vi "Sensor - Find theta and position - shih.vi"() -> ()   [LabVIEW 2016]
uses:
  Classes/Controllers/Motion/Copy of Motion Folder/Motion.lvclass
  Classes/Controllers/Camera/Copy of Controller Folder/Controller.lvclass
panel:
  out "Type B rotation error":dbl format="%#_8e"
  out "Type B Y error":dbl format="%#_8g"
  out "Type B X error":dbl format="%#_8g"
  out "Type A rotation error":dbl format="%#_8e"
  out "Type A Y error":dbl format="%#_8g"
  out "Type A X error":dbl format="%#_8g"
  in  "position A":dbl[](array[numeric])=[450.0333, 1074.4422, 78.966399, 0.019289062] format="%#_10g"
  in  "Boolean":bool
  out "HDI/sesnor array":bool[](array[boolean])
  out "type a/b array":bool[](array[boolean])
  in  "C 2":dbl[](array[numeric])=[322.268517526742, 1153.5721313313948, 79.00539576014785, 0.01961841234863117] format="%#_10g"
  in  "B 2":dbl[](array[numeric])=[300.2655109951287, 1153.8313815706124, 79.00573186765678, 0.019288904062814086] format="%#_10g"
  in  "position A 2":dbl[](array[numeric])=[299.0519921586575, 1052.343019098103, 79.00564961071272, 0.019294304149470937] format="%#_10g"
  in  "C":dbl[](array[numeric])=[475.67567, 1203.3475, 78.955395, 0.019618489] format="%#_10g"
  in  "B":dbl[](array[numeric])=[451.38655, 1203.5959, 78.956401, 0.019289062] format="%#_10g"
  in  "position A 4":dbl[](array[numeric])=[299.0519921586575, 1052.343019098103, 79.00564961071272, 0.019294304149470937] format="%#_10g"
  in  "B 4":dbl[](array[numeric])=[300.2655109951287, 1153.8313815706124, 79.00573186765678, 0.019288904062814086] format="%#_10g"
  in  "C 4":dbl[](array[numeric])=[322.268517526742, 1153.5721313313948, 79.00539576014785, 0.01961841234863117] format="%#_10g"
  in  "position A 3":dbl[](array[numeric])=[450.75355, 1073.8809, 78.571159, 0.019294304149470937] format="%#_10g"
  in  "B 3":dbl[](array[numeric])=[452.11281, 1203.3722, 78.624175, 0.019288904062814086] format="%#_10g"
  in  "C 3":dbl[](array[numeric])=[474.11351, 1203.144, 78.625406, 0.01961841234863117] format="%#_10g"
  in  "Type A/ Type B":bool
  in  "HDI / Sensor":bool
  out "the copy array":dbl[](array[numeric]) format="%#_8g"
  out "buttom right C":dbl[](array[numeric]) format="%#_8g"
  out "X position":dbl[](array[numeric]) format="%#_8g"
  out "Yposition":dbl[](array[numeric]) format="%#_8g"
  out "A C center point":dbl[](array[numeric]) format="%#_8g"
  out "counting":dbl
  out "rotation":dbl[](array[numeric]) format="%#_8g"
  in  "Parking position":dbl[](array[numeric])=[625.0, 625.0, 0.0, 0.01]
  in  "Stop":bool
  in  "DO measurement":bool=TRUE
  out "buttom left B":dbl[](array[numeric]) format="%#_8g"
  out "upper left A":dbl[](array[numeric]) format="%#_8g"
  out "r-phi":dbl[](array[numeric])
  out "A B center point":dbl[](array[numeric])
  # "HDI"
  # "type A"
  # "Sensor"
  # "type B"
  # "type A"
  # "type B"
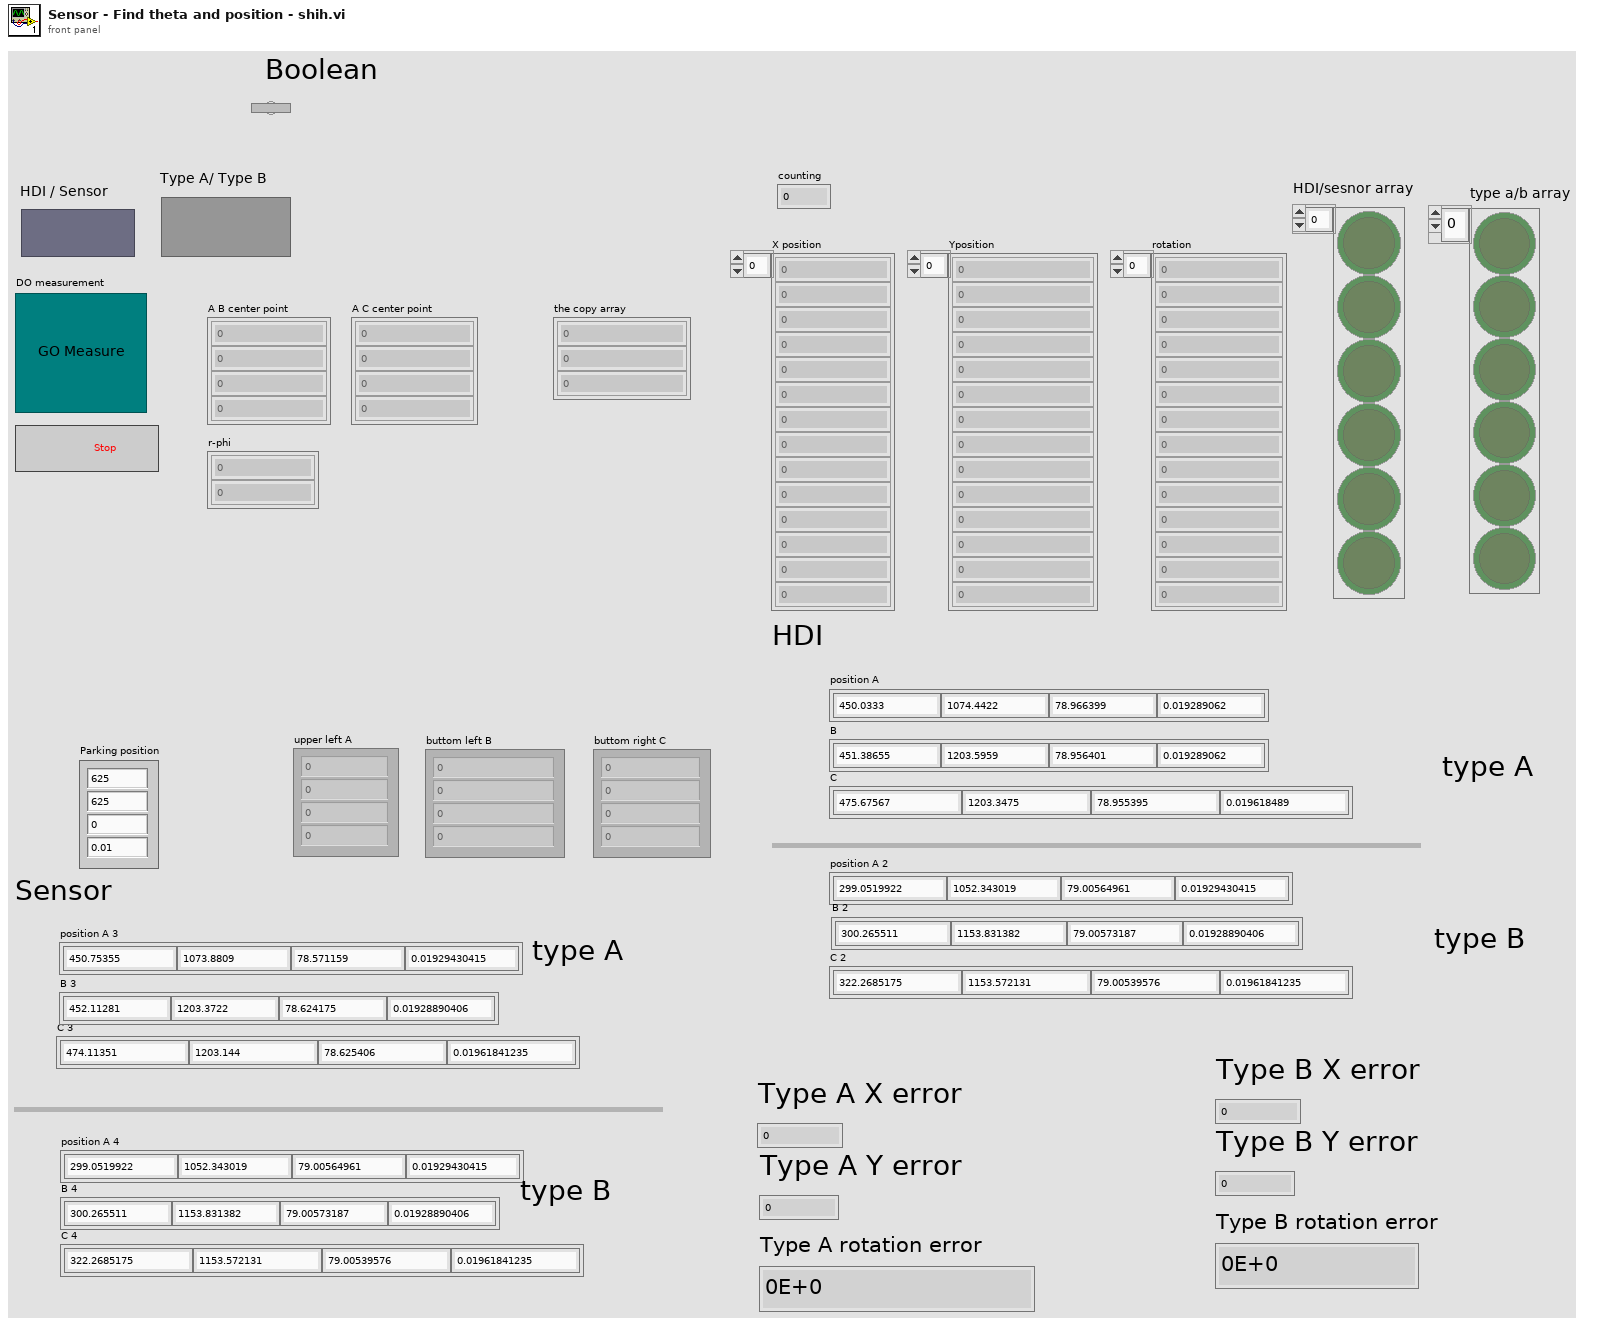
[diagram p1: front panel]
types:
  T1 = typedef "Controller.lvclass/Controllers.ctl" = cluster{"Copy of Motion.lvclass":refnum<class "Motion.lvclass">, "Copy of I-O.lvclass":refnum<class "I-O.lvclass">, "Copy of Dispenser.lvclass":refnum<class "Dispenser.lvclass">}
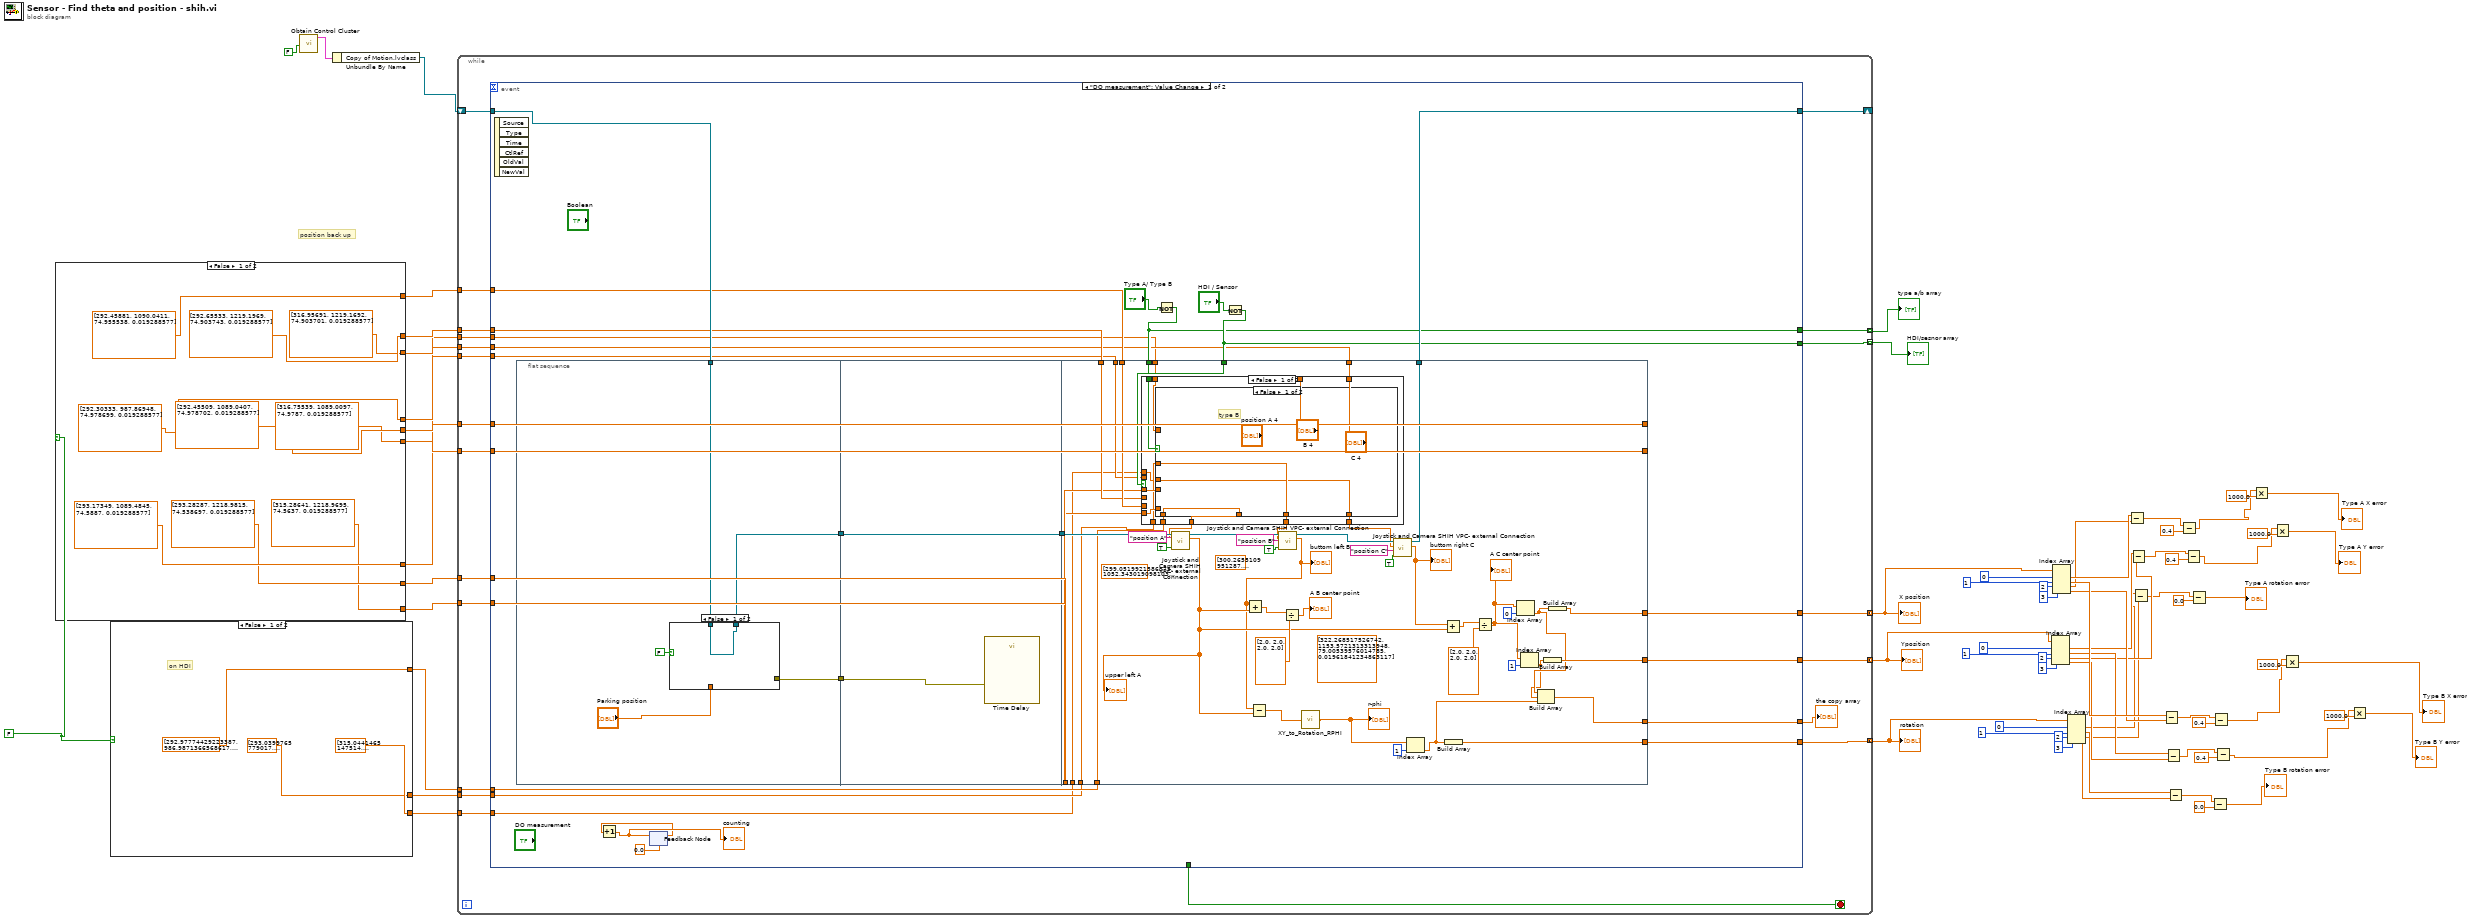
[diagram p0: block diagram]
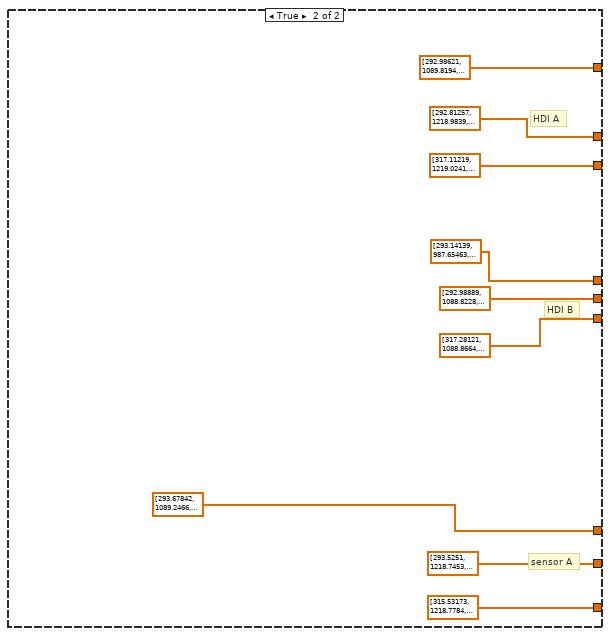
[diagram p2: hidden frame]
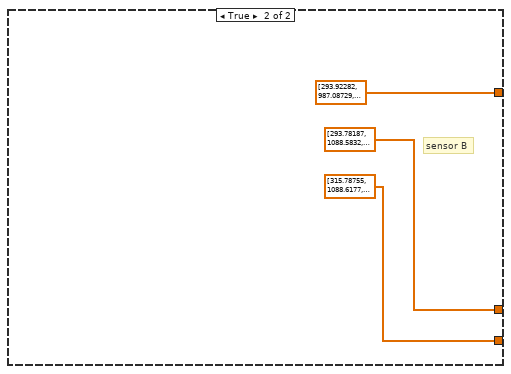
[diagram p3: hidden frame]
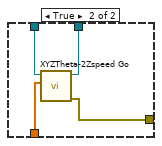
[diagram p4: hidden frame]
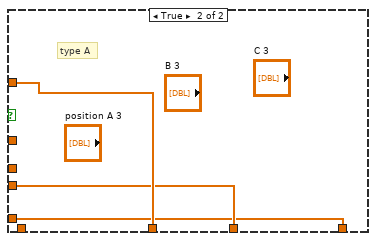
[diagram p5: hidden frame]
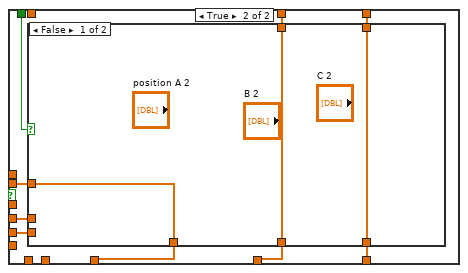
[diagram p6: hidden frame]
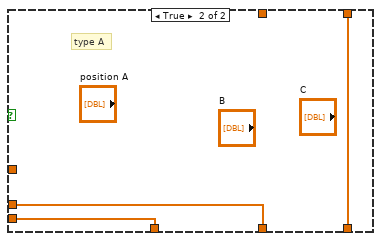
[diagram p7: hidden frame]
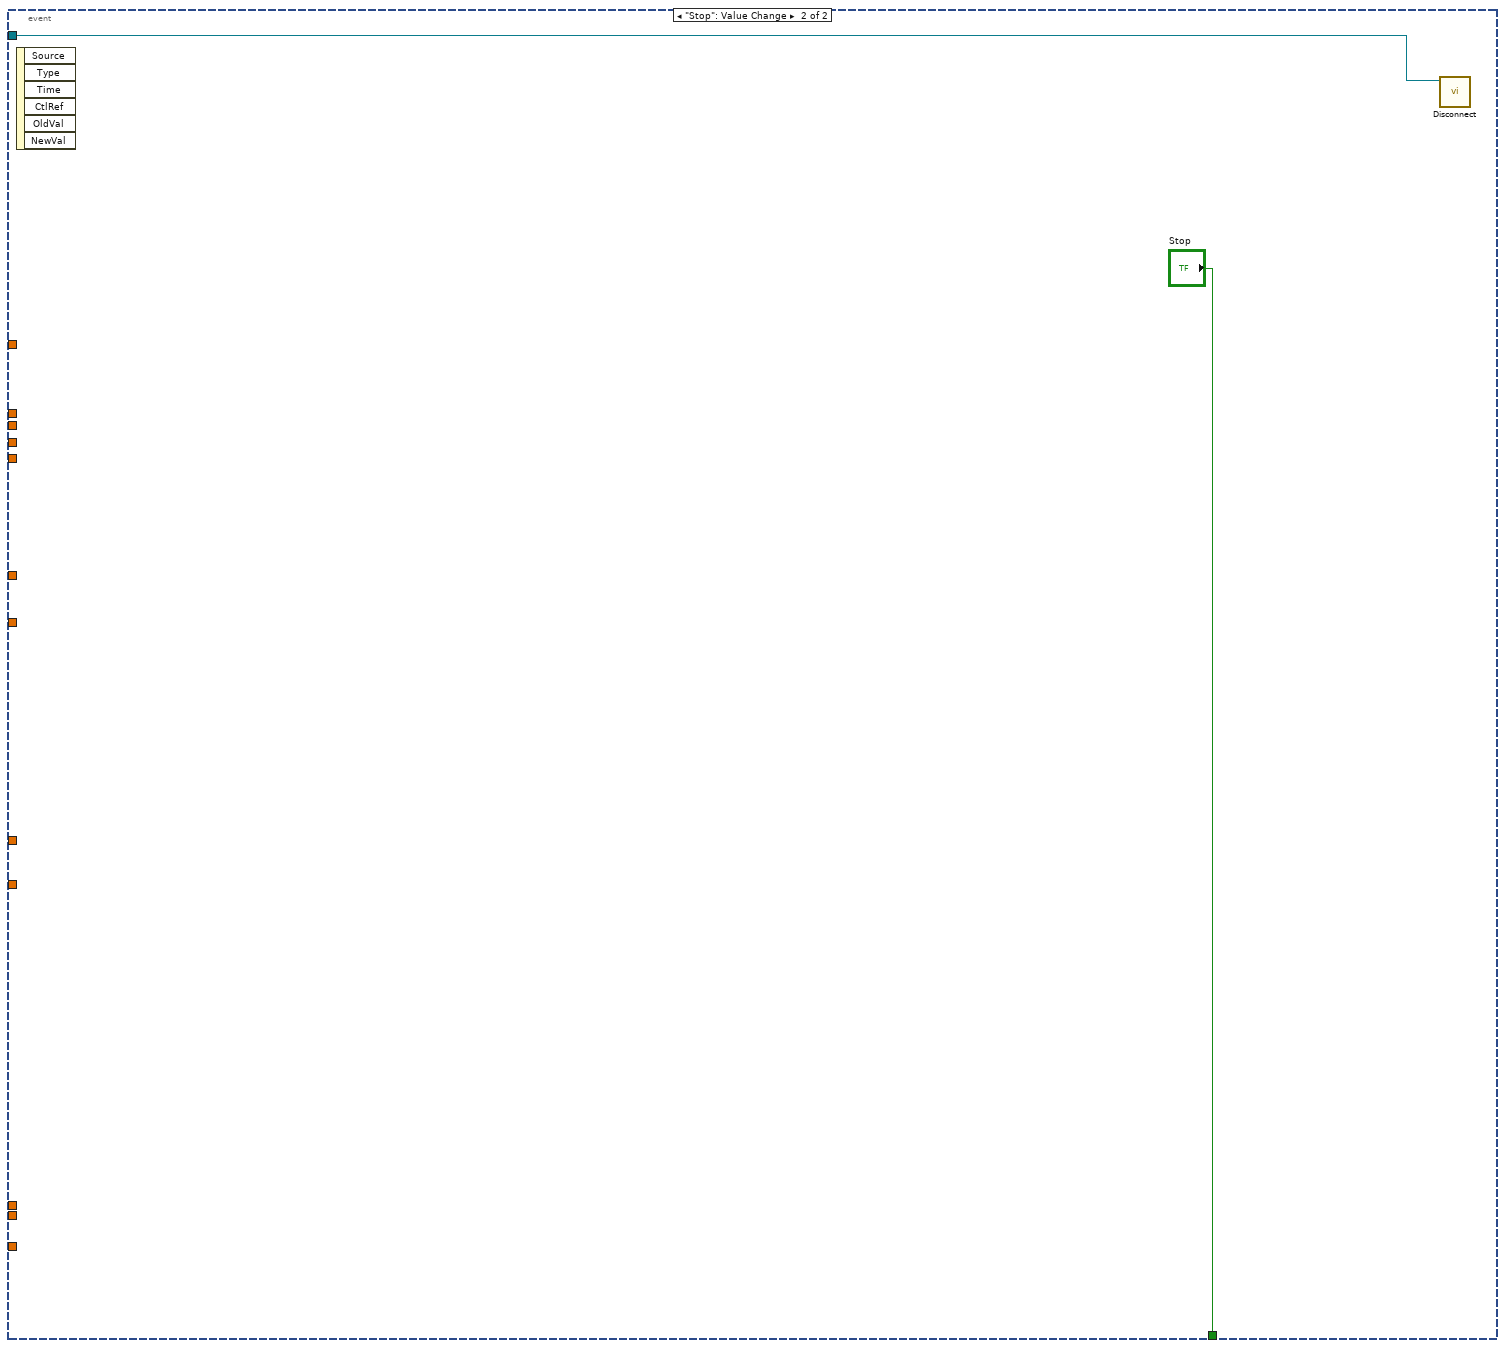
[diagram p8: hidden frame]
diagram:
  w1 = FALSE
  # "position back up"
  n1 = case shown="False" w1 {
    tunnel: [dbl[] [292.45881, 1090.0411, 74.955538, 0.019288577] dbl[] [292.98621, 1089.8194, 78.916401, 0.019289062] ("position A")] -> w66
    tunnel: [dbl[] [292.65533, 1219.1969, 74.903743, 0.019288577] dbl[] [292.81257, 1218.9839, 78.916401, 0.019289062] ("B")] -> w65
    tunnel: [dbl[] [316.95691, 1219.1692, 74.903701, 0.019288577] dbl[] [317.11219, 1219.0241, 78.955395, 0.019618489] ("C")] -> w64
    tunnel: [dbl[] [292.30333, 987.86948, 74.978699, 0.019288577] dbl[] [293.14139, 987.65463, 79.00564961071272, 0.019294304149470937] ("position A 2")] -> w63
    tunnel: [dbl[] [292.45509, 1089.0407, 74.978702, 0.019288577] dbl[] [292.98889, 1088.8228, 79.00573186765678, 0.019288904062814086] ("B 2")] -> w62
    tunnel: [dbl[] [316.75539, 1089.0097, 74.9787, 0.019288577] dbl[] [317.28121, 1088.8664, 79.00539576014785, 0.01961841234863117] ("C 2")] -> w61
    tunnel: [dbl[] [293.17349, 1089.4845, 74.5887, 0.019288577] dbl[] [293.67842, 1089.2466, 79.00564961071272, 0.019294304149470937] ("position A 3")] -> w60
    tunnel: [dbl[] [293.28287, 1218.9815, 74.538697, 0.019288577] dbl[] [293.5251, 1218.7453, 79.00573186765678, 0.019288904062814086] ("B 3")] -> w59
    tunnel: [dbl[] [315.28641, 1218.9695, 74.5637, 0.019288577] dbl[] [315.53173, 1218.7784, 79.00539576014785, 0.01961841234863117] ("C 3")] -> w58
    frame False {
    }
    frame True {
      # "sensor A"
      # "HDI B"
      # "HDI A"
    }
  }
  n2 = case shown="False" w1 {
    tunnel: [dbl[] [292.97774429223387, 986.9871366568617, 74.58809514732275, 0.01929431396256771] ("upper left A") dbl[] [293.92282, 987.08729, 79.00564961071272, 0.019294304149470937] ("position A 4")] -> w57
    tunnel: [dbl[] [293.0399765779017, 1088.4809837209998, 74.5881025119211, 0.019289091243472195] ("buttom left B") dbl[] [293.78187, 1088.5832, 79.00573186765678, 0.019288904062814086] ("B 4")] -> w56
    tunnel: [dbl[] [315.0441465147514, 1088.473568846111, 74.56310054097365, 0.019618446130758856] ("buttom right C") dbl[] [315.78755, 1088.6177, 79.00539576014785, 0.01961841234863117] ("C 4")] -> w55
    frame False {
      # "on HDI"
    }
    frame True {
      # "sensor B"
    }
  }
  n3 = call "Obtain Control Cluster.vi"("I/O"=FALSE) -> ("Control Out"=w71:T1)  [unwired: 10 in]
  n4 = Unbundle By Name(w71) -> ("Copy of Motion.lvclass"=w69:refnum<class "Motion.lvclass">)
  n5 = while {
    shift-right: [w114] -> _
    shift-left: w69 -> [w116]
    tunnel: [w113] -> w40 mode=concatenating
    tunnel: [w112] -> w42 mode=concatenating
    tunnel: [w111] -> w41 mode=concatenating
    tunnel: [w109] -> w68 mode=indexing
    tunnel: [w108] -> w67 mode=indexing
    tunnel: w66 -> [w107]
    tunnel: w65 -> [w106]
    tunnel: w64 -> [w105]
    tunnel: w63 -> [w104]
    tunnel: w62 -> [w103]
    tunnel: w61 -> [w102]
    tunnel: w60 -> [w101]
    tunnel: w59 -> [w100]
    tunnel: w58 -> [w99]
    tunnel: w57 -> [w98]
    tunnel: w56 -> [w97]
    tunnel: w55 -> [w96]
    stop <- w115 stop-if-true
    n6 = event shown="[0] \"DO measurement\": Value Change" {
      selector: _ -> [_ _]
      dyn-events: _ -> [_ _]
      timeout: _ -> [_ _]
      tunnel: w116 -> [w144 w238]
      tunnel: [_ "Stop"] -> w115
      tunnel: [w139 _] -> w114
      tunnel: [w140 _] -> w113
      tunnel: [w135 _] -> w112
      tunnel: [w134 _] -> w111
      tunnel: [w133 _] -> w110
      tunnel: [w129 _] -> w109
      tunnel: [w131 _] -> w108
      tunnel: w107 -> [w128 _]
      tunnel: w106 -> [w127 _]
      tunnel: w105 -> [w126 _]
      tunnel: w104 -> [w125 _]
      tunnel: w103 -> [w124 _]
      tunnel: w102 -> [w123 _]
      tunnel: w101 -> [w122 _]
      tunnel: w100 -> [w121 _]
      tunnel: w99 -> [w120 _]
      tunnel: w98 -> [w119 _]
      tunnel: w97 -> [w118 _]
      tunnel: w96 -> [w117 _]
      event "DO measurement": Value Change {
        n7 = event-data() -> ()  [unwired: 1 in, 6 out]
        n8 = flat-sequence {
          tunnel: w144 -> [w148]
          tunnel: [w147] -> w143
          tunnel: [w146] -> w141
          tunnel: w143 -> [w156]
          tunnel: [w155] -> w142
          tunnel: w141 -> [w155]
          tunnel: w142 -> [w197]
          tunnel: [w194] -> w140
          tunnel: [w191] -> w139
          tunnel: [w184] -> w135
          tunnel: [w183] -> w134
          tunnel: [w176] -> w133
          tunnel: w131 -> [w175]
          tunnel: w129 -> [w174]
          tunnel: w128 -> [w170]
          tunnel: w127 -> [w169]
          tunnel: w126 -> [w168]
          tunnel: w125 -> [w167]
          tunnel: w124 -> [w166]
          tunnel: w123 -> [w165]
          tunnel: w122 -> [w164]
          tunnel: w121 -> [w163]
          tunnel: w120 -> [w162]
          tunnel: w119 -> [w161]
          tunnel: w118 -> [w160]
          tunnel: w117 -> [w159]
          frame #0 {
            n9 = case shown="False" FALSE {
              tunnel: "Parking position" -> [_ w154]
              tunnel: w148 -> [w150 w153]
              tunnel: [_ w152] -> w147
              tunnel: [w150 w151] -> w146
              frame False {
              }
              frame True {
                n10 = call "XYZTheta-2Zspeed Go.vi"("XYZTheta In"=w154, "Motion in"=w153) -> ("error out"=w152:errorcluster, "Motion out"=w151:refnum<class "Motion.lvclass">)  [unwired: 7 in, 1 out]
              }
            }
          }
          frame #1 {
            n11 = call "Time Delay"("error in (no error)"=w156) -> ()  [unwired: 10 in, 1 out]
          }
          frame #2 {
            (unwired) dbl[] [322.268517526742, 1153.5721313313948, 79.00539576014785, 0.01961841234863117] ("Gantry")
            (unwired) dbl[] [300.2655109951287, 1153.8313815706124, 79.00573186765678, 0.019288904062814086] ("Sum")
            (unwired) dbl[] [299.0519921586575, 1052.343019098103, 79.00564961071272, 0.019294304149470937] ("Sum")
            n12 = case shown="False" w175 {
              tunnel: w174 -> [w214 w230]
              tunnel: [w213 w229] -> w173
              tunnel: [w212 w228] -> w172
              tunnel: [w211 w227] -> w171
              tunnel: w170 -> [_ w226]
              tunnel: w169 -> [_ w225]
              tunnel: w168 -> [_ w224]
              tunnel: w167 -> [_ w223]
              tunnel: w166 -> [_ w222]
              tunnel: w165 -> [_ w221]
              tunnel: w164 -> [w210 _]
              tunnel: w163 -> [w209 _]
              tunnel: w162 -> [w208 _]
              tunnel: w161 -> [w207 _]
              tunnel: w160 -> [w206 _]
              tunnel: w159 -> [w205 _]
              frame False {
                n13 = case shown="False" w214 {
                  tunnel: [w217 w220] -> w213
                  tunnel: [w216 w219] -> w212
                  tunnel: [w215 w218] -> w211
                  tunnel: w210 -> [_ w220]
                  tunnel: w209 -> [_ w219]
                  tunnel: w208 -> [_ w218]
                  tunnel: w207 -> [w217 _]
                  tunnel: w206 -> [w216 _]
                  tunnel: w205 -> [w215 _]
                  frame False {
                    # "type B"
                  }
                  frame True {
                    # "type A"
                  }
                }
              }
              frame True {
                n14 = case shown="False" w230 {
                  tunnel: [w233 w236] -> w229
                  tunnel: [w232 w235] -> w228
                  tunnel: [w231 w234] -> w227
                  tunnel: w226 -> [_ w236]
                  tunnel: w225 -> [_ w235]
                  tunnel: w224 -> [_ w234]
                  tunnel: w223 -> [w233 _]
                  tunnel: w222 -> [w232 _]
                  tunnel: w221 -> [w231 _]
                  frame False {
                  }
                  frame True {
                    # "type A"
                  }
                }
              }
            }
            n15 = call "Joystick and Camera SHIH VPC- external Connection.vi"("Motion in"=w197, "XYZTheta"=w173, "Measurement Point"="position A", "Inital GO"=TRUE) -> ("Motion out"=w200:refnum<class "Motion.lvclass">, "Sum"=w158:dbl[])  [unwired: 3 in, 2 out]
            "upper left A" <- w158
            n16 = call "Joystick and Camera SHIH VPC- external Connection.vi"("Motion in"=w200, "XYZTheta"=w172, "Measurement Point"="position B", "Inital GO"=TRUE) -> ("Motion out"=w192:refnum<class "Motion.lvclass">, "Sum"=w157:dbl[])  [unwired: 3 in, 2 out]
            "buttom left B" <- w157
            n17 = Add(x=w157, y=w158) -> (x+y=w201:dbl[])
            n18 = Subtract(x=w157, y=w158) -> (x-y=w204:dbl[])
            n19 = Divide(x=w201, y=dbl[] [2.0, 2.0, 2.0, 2.0]) -> (x/y=→"A B center point":dbl[])
            n20 = call "XY_to_Rotation_RPHI.vi"("X-Y"=w204) -> ("r-phi"=w195:dbl[])
            "r-phi" <- w195
            n21 = call "Joystick and Camera SHIH VPC- external Connection.vi"("Motion in"=w192, "XYZTheta"=w171, "Measurement Point"="position C", "Inital GO"=TRUE) -> ("Motion out"=w191:refnum<class "Motion.lvclass">, "Sum"=w190:dbl[])  [unwired: 3 in, 2 out]
            "buttom right C" <- w190
            n22 = Index Array(array=w195, index=1) -> (element=w180:dbl)
            n23 = Add(x=w190, y=w158) -> (x+y=w188:dbl[])
            n24 = Build Array(w180) -> (w194:dbl[])
            n25 = Divide(x=w188, y=dbl[] [2.0, 2.0, 2.0, 2.0]) -> (x/y=w185:dbl[])
            "A C center point" <- w185
            n26 = Index Array(array=w185, index=0) -> (element=w182:dbl)
            n27 = Index Array(array=w185, index=1) -> (element=w181:dbl)
            n28 = Build Array(w182, w181, w180) -> (w176:dbl[])
            n29 = Build Array(w181) -> (w183:dbl[])
            n30 = Build Array(w182) -> (w184:dbl[])
          }
        }
        n31 = feedback #1(0.0) -> (w136:dbl)
        n32 = Increment(x=w136) -> (x+1=w138:dbl)
        "counting" <- w138
        n33 = feedback-in #1(w138) -> ()
        n34 = Not(x="Type A/ Type B") -> (.not. x?=w129:bool)
        n35 = Not(x="HDI / Sensor") -> (.not. x?=w131:bool)
      }
      event "Stop": Value Change {
        n36 = event-data() -> ()  [unwired: 1 in, 6 out]
        n37 = call-dynamic "Disconnect.vi"("Controller in"=w238) -> ()  [unwired: 9 in, 1 out]
      }
    }
    "the copy array" <- w110
  }
  "rotation" <- w40
  "X position" <- w42
  "Yposition" <- w41
  "type a/b array" <- w68
  "HDI/sesnor array" <- w67
  n38 = Index Array(array=w41, index #1=0 ("index"), index #2=1 ("index"), index #3=2 ("index"), index #4=3 ("index")) -> (element #1=w35:dbl, element #2=w34:dbl, element #3=w33:dbl, element #4=w32:dbl)
  n39 = Index Array(array=w42, index #1=0 ("index"), index #2=1 ("index"), index #3=2 ("index"), index #4=3 ("index")) -> (element #1=w39:dbl, element #2=w38:dbl, element #3=w37:dbl, element #4=w36:dbl)
  n40 = Index Array(array=w40, index #1=0 ("index"), index #2=1 ("index"), index #3=2 ("index"), index #4=3 ("index")) -> (element #1=w31:dbl, element #2=w30:dbl, element #3=w29:dbl, element #4=w28:dbl)
  n41 = Subtract(x=w39, y=w37) -> (x-y=w21:dbl)
  n42 = Subtract(x=w35, y=w33) -> (x-y=w20:dbl)
  n43 = Subtract(x=w31, y=w29) -> (x-y=w19:dbl)
  n44 = Subtract(x=w38, y=w36) -> (x-y=w18:dbl)
  n45 = Subtract(x=w34, y=w32) -> (x-y=w17:dbl)
  n46 = Subtract(x=w30, y=w28) -> (x-y=w16:dbl)
  n47 = Subtract(x=w21, y=0.4) -> (x-y=w12:dbl)
  n48 = Subtract(x=w20, y=0.4) -> (x-y=w9:dbl)
  n49 = Subtract(x=w19, y=0.0) -> (x-y=→"Type A rotation error":dbl)
  n50 = Subtract(x=w16, y=0.0) -> (x-y=→"Type B rotation error":dbl)
  n51 = Subtract(x=w18, y=0.4) -> (x-y=w6:dbl)
  n52 = Subtract(x=w17, y=0.4) -> (x-y=w3:dbl)
  n53 = Multiply(x=w12, y=1000.0) -> (x*y=→"Type A X error":dbl)
  n54 = Multiply(x=w9, y=1000.0) -> (x*y=→"Type A Y error":dbl)
  n55 = Multiply(x=w6, y=1000.0) -> (x*y=→"Type B X error":dbl)
  n56 = Multiply(x=w3, y=1000.0) -> (x*y=→"Type B Y error":dbl)
